vi "Open VI as Dialog.vi"(8 "error in (no error)":errorcluster, 10 "This Application":refnum<vi>, 11 "VI in":refnum<vi>) -> (0 "error out":errorcluster)   [LabVIEW 2013, in "OPC UA editor node.lvclass"]
uses:
  OPC UA editor node.lvclass
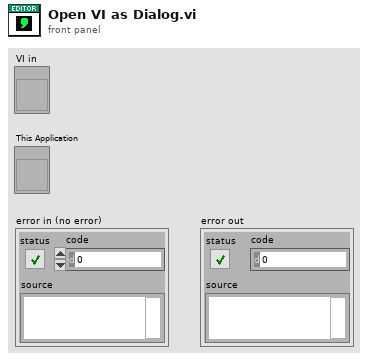
[diagram p1: front panel]
types:
  T1 = enum32{"Invalid", "Standard", "Closed", "Hidden", "Minimized", "Maximized"}
  T2 = enum32{"invalid app kind", "Development System", "Run Time System", "Student Edition", "Embedded LabVIEW", "Evaluation", "Custom"}
  T3 = enum32{"Invalid", "Default", "Floating", "Floating/Auto-Hide", "Modal"}
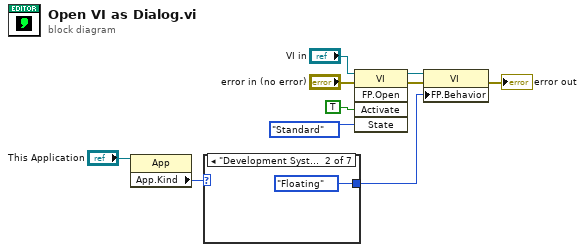
[diagram p0: block diagram]
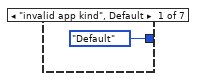
[diagram p2: hidden frame]
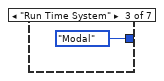
[diagram p3: hidden frame]
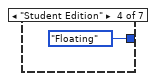
[diagram p4: hidden frame]
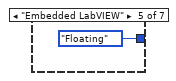
[diagram p5: hidden frame]
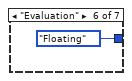
[diagram p6: hidden frame]
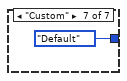
[diagram p7: hidden frame]
diagram:
  n1 = property class="App"(reference="This Application") -> ("App.Kind"=w2:T2)  [unwired: 1 in, 2 out]
  n2 = case shown="\"Development System\"" w2 {
    tunnel: [T3."Default" ("Front Panel Window:Behavior") T3."Floating" ("Front Panel Window:Behavior") T3."Modal" ("Front Panel Window:Behavior") T3."Floating" ("Front Panel Window:Behavior") T3."Floating" ("Front Panel Window:Behavior") T3."Floating" ("Front Panel Window:Behavior") T3."Default" ("Front Panel Window:Behavior")] -> w1
    frame "invalid app kind", Default {
    }
    frame "Development System" {
    }
    frame "Run Time System" {
    }
    frame "Student Edition" {
    }
    frame "Embedded LabVIEW" {
    }
    frame "Evaluation" {
    }
    frame "Custom" {
    }
  }
  n3 = invoke class="VI" method="FP.Open"(reference="VI in", error in="error in (no error)", "Activate"=TRUE ("Activate?"), "State"=T1."Standard") -> (reference out=w7:refnum<vi>, error out=w8:errorcluster)  [unwired: 1 in, 3 out]
  n4 = property class="VI"(reference=w7, error in=w8, "FP.Behavior"=w1) -> (error out=→"error out":errorcluster)  [unwired: 1 out]
